vi "BMU诊断标定.vi"(5 "timeout":u32, 6 "Socket":dbl, 7 "通用配置?":bool, 8 "CAN端口":u16(ring), 9 "设备索引号":u16(ring), 10 "CAN卡类型":u32(ring)=21, 11 "从板号":u8=1) -> (3 "成功?":bool)   [LabVIEW 2013] (continued)
                                frame "电压起始值" {
                                n3880 = disable-structure shown="禁用" {
                                frame Disabled {
                                n3881 = local read "从板个数"() -> (w5557:dbl)
                                n3882 = Increment(x=w5557) -> (x+1=w5556:dbl)
                                n3883 = control-ref of="项目信息"() -> (w5563:refnum<vi>)
                                n3884 = for {
                                N: w5556 -> [_]
                                tunnel: [""] -> w5562 mode=indexing
                                }
                                n3885 = Multiply(x=u8 1, y=w5557) -> (x*y=w5559:dbl)
                                n3886 = Add(x=w5559, y=u8 21) -> (x+y=w5555:dbl)
                                n3887 = call "表格数据输入-8.6.vi"("行数"=w5555, "列数"=u32 1, "字符串数组"=w5562, "表格引用"=w5563) -> ()  [unwired: 8 in]
                                }
                                frame Enabled {
                                }
                                }
                                }
                                frame "温度个数" {
                                n3888 = local read "从板个数"() -> (w5567:dbl)
                                n3889 = Increment(x=w5567) -> (x+1=w5566:dbl)
                                n3890 = control-ref of="项目信息"() -> (w5573:refnum<vi>)
                                n3891 = for {
                                N: w5566 -> [_]
                                tunnel: [""] -> w5572 mode=indexing
                                }
                                n3892 = Multiply(x=u8 2, y=w5567) -> (x*y=w5569:dbl)
                                n3893 = Add(x=w5569, y=u8 22) -> (x+y=w5565:dbl)
                                n3894 = call "表格数据输入-8.6.vi"("行数"=w5565, "列数"=u32 1, "字符串数组"=w5572, "表格引用"=w5573) -> ()  [unwired: 8 in]
                                }
                                frame "温度起始值" {
                                n3895 = disable-structure shown="禁用" {
                                frame Disabled {
                                n3896 = local read "从板个数"() -> (w5577:dbl)
                                n3897 = Increment(x=w5577) -> (x+1=w5576:dbl)
                                n3898 = control-ref of="项目信息"() -> (w5583:refnum<vi>)
                                n3899 = for {
                                N: w5576 -> [_]
                                tunnel: [""] -> w5582 mode=indexing
                                }
                                n3900 = Multiply(x=u8 3, y=w5577) -> (x*y=w5579:dbl)
                                n3901 = Add(x=w5579, y=u8 23) -> (x+y=w5575:dbl)
                                n3902 = call "表格数据输入-8.6.vi"("行数"=w5575, "列数"=u32 1, "字符串数组"=w5582, "表格引用"=w5583) -> ()  [unwired: 8 in]
                                }
                                frame Enabled {
                                }
                                }
                                }
                                frame "保险位置" {
                                n3903 = local read "从板个数"() -> (w5587:dbl)
                                n3904 = control-ref of="项目信息"() -> (w5593:refnum<vi>)
                                n3905 = for {
                                N: 10 -> [_]
                                tunnel: [""] -> w5592 mode=indexing
                                }
                                n3906 = Multiply(x=u8 4, y=w5587) -> (x*y=w5589:dbl)
                                n3907 = Add(x=w5589, y=u8 24) -> (x+y=w5586:dbl)
                                n3908 = call "表格数据输入-8.6.vi"("行数"=w5586, "列数"=u32 1, "字符串数组"=w5592, "表格引用"=w5593) -> ()  [unwired: 8 in]
                                }
                                frame "电池额定实际容量" {
                                w5595 = 0.0 ("值")
                                n3909 = control-ref of="电池实际容量(A)"() -> (w5596:refnum<vi>)
                                n3910 = control-ref of="电池额定容量(A)"() -> (w5597:refnum<vi>)
                                n3911 = property class="DigNum (严格)"(reference=w5596, "Value"=w5595) -> ()  [unwired: 1 in, 2 out]
                                n3912 = property class="DigNum (严格)"(reference=w5597, "Value"=w5595) -> ()  [unwired: 1 in, 2 out]
                                }
                                frame "SOC" {
                                n3913 = control-ref of="SOC(%)"() -> (w5598:refnum<vi>)
                                n3914 = property class="DigNum (严格)"(reference=w5598, "Value"=0.0 ("值")) -> ()  [unwired: 1 in, 2 out]
                                }
                                frame "配置文件版本" {
                                n3915 = control-ref of="配置文件版本"() -> (w5600:refnum<vi>)
                                n3916 = property class="Str"(reference=w5600, "Value"="" ("值")) -> ()  [unwired: 1 in, 2 out]
                                }
                                frame "参数修改记录" {
                                n3917 = control-ref of="使用者"() -> (w5603:refnum<vi>)
                                n3918 = control-ref of="系统时钟"() -> (w5604:refnum<vi>)
                                n3919 = property class="DigNum (严格)"(reference=w5603, "Value"=0.0 ("值")) -> ()  [unwired: 1 in, 2 out]
                                n3920 = property class="Str"(reference=w5604, "Value"="" ("值")) -> ()  [unwired: 1 in, 2 out]
                                }
                                frame "校正时钟" {
                                n3921 = control-ref of="系统时钟"() -> (w5606:refnum<vi>)
                                n3922 = property class="Str"(reference=w5606, "Value"="" ("值")) -> ()  [unwired: 1 in, 2 out]
                                }
                                frame "车牌号" {
                                n3923 = control-ref of="车架(牌)号"() -> (w5608:refnum<vi>)
                                n3924 = property class="Str"(reference=w5608, "Value"="" ("值")) -> ()  [unwired: 1 in, 2 out]
                                }
                                frame "SOH" {
                                n3925 = control-ref of="SOH(%)"() -> (w5611:refnum<vi>)
                                n3926 = property class="DigNum (严格)"(reference=w5611, "Value"=0.0 ("值")) -> ()  [unwired: 1 in, 2 out]
                                }
                                frame "一级故障阀值" {
                                n3927 = local write "一级故障"(T10 {"总电压过高"=0.0, "整组电压不均衡"=0.0, "SOC过高"=0.0, "单体电压过高"=0.0, "总电压过低"=0.0, "温度过高"=0.0, "温度过低"=0.0, "单组电压不均衡"=0.0, "整组温度不均衡"=0.0, "单组温度不均衡"=0.0, "单体电压过低"=0.0, "充电电流过高"=0.0, "放电电流过高"=0.0, "SOC过低"=0.0, "内阻过大"=0.0, "极柱温度过高"=0.0, "SOH过低"=0.0} ("一级故障")) -> ()
                                }
                                frame "二级故障阀值" {
                                n3928 = local write "一级故障 2"(T10 {"总电压过高"=0.0, "整组电压不均衡"=0.0, "SOC过高"=0.0, "单体电压过高"=0.0, "总电压过低"=0.0, "温度过高"=0.0, "温度过低"=0.0, "单组电压不均衡"=0.0, "整组温度不均衡"=0.0, "单组温度不均衡"=0.0, "单体电压过低"=0.0, "充电电流过高"=0.0, "放电电流过高"=0.0, "SOC过低"=0.0, "内阻过大"=0.0, "极柱温度过高"=0.0, "SOH过低"=0.0} ("一级故障")) -> ()
                                }
                                frame "三级故障阀值" {
                                n3929 = local write "一级故障 3"(T10 {"总电压过高"=0.0, "整组电压不均衡"=0.0, "SOC过高"=0.0, "单体电压过高"=0.0, "总电压过低"=0.0, "温度过高"=0.0, "温度过低"=0.0, "单组电压不均衡"=0.0, "整组温度不均衡"=0.0, "单组温度不均衡"=0.0, "单体电压过低"=0.0, "充电电流过高"=0.0, "放电电流过高"=0.0, "SOC过低"=0.0, "内阻过大"=0.0, "极柱温度过高"=0.0, "SOH过低"=0.0} ("一级故障")) -> ()
                                }
                                frame "加热控制参数" {
                                n3930 = local write "加热控制参数"(T11 {"风机开启温度"=0.0, "风机关闭温度"=0.0, "加热开启温度"=0.0, "加热关闭温度"=0.0, "风机开启温差"=0.0, "风机关闭温差"=0.0, "加热关闭温差"=0.0} ("加热控制参数")) -> ()
                                }
                                frame "充电控制参数" {
                                n3931 = local write "一级故障 5"(T12 {"最大允许单体电压"=0.0, "最大允许总电压"=0.0, "最小允许单体电压"=0.0, "最大允许充电电流"=0.0, "最小允许充电电流"=0.0, "最大允许充电温度"=0.0, "最小允许充电温度"=0.0, "电流步长"=0.0} ("一级故障 5")) -> ()
                                }
                                frame "电池信息1" {
                                w5617 = ""
                                w5618 = 0.0 ("电池串联")
                                n3932 = local read "电池信息"() -> (w5620:T13)
                                n3933 = Bundle By Name(cluster=w5620, "电池串联"=w5618, "电池并联"=w5618, "电池包额定容量"=w5618, "电池包额定能量(kWh)"=w5618, "电池包额定总电压"=w5618, "实际容量"=w5618, "电池厂家"=w5617, "电池类型"=w5617, "电池生产日期"=w5617) -> (w5619:T13)
                                n3934 = local write "电池信息"(w5619) -> ()
                                }
                                frame "电池包组号" {
                                n3935 = local read "电池信息"() -> (w5623:T13)
                                n3936 = Bundle By Name(cluster=w5623, "电池包组号"="") -> (w5622:T13)
                                n3937 = local write "电池信息"(w5622) -> ()
                                }
                                frame "充放电安时" {
                                w5624 = 0.0 ("累计充电总安时")
                                n3938 = local read "电池信息"() -> (w5626:T13)
                                n3939 = Bundle By Name(cluster=w5626, "累计充电总安时"=w5624, "累计放电总安时"=w5624) -> (w5625:T13)
                                n3940 = local write "电池信息"(w5625) -> ()
                                }
                                frame "电池充放电次数" {
                                w5627 = 0.0 ("累计充电总安时")
                                n3941 = local read "电池信息"() -> (w5629:T13)
                                n3942 = Bundle By Name(cluster=w5629, "电池充满次数"=w5627, "电池放空次数"=w5627, "电池充电次数"=w5627) -> (w5628:T13)
                                n3943 = local write "电池信息"(w5628) -> ()
                                }
                                }
                              }
                              frame "从板" {
                                n3944 = case shown="\"温度起始值\"" w5630 {
                                frame "假", Default {
                                }
                                frame "电压起始值" {
                                n3945 = for {
                                N: 1 -> [_]
                                tunnel: [""] -> w5635 mode=indexing
                                }
                                n3946 = control-ref of="项目信息 2"() -> (w5631:refnum<vi>)
                                n3947 = call "表格数据输入-8.6.vi"("行数"=u32 0, "列数"=u32 1, "字符串数组"=w5635, "表格引用"=w5631) -> ()  [unwired: 8 in]
                                }
                                frame "通道电压个数" {
                                n3948 = for {
                                N: 5 -> [_]
                                tunnel: [""] -> w5641 mode=indexing
                                }
                                n3949 = control-ref of="项目信息 2"() -> (w5637:refnum<vi>)
                                n3950 = call "表格数据输入-8.6.vi"("行数"=u32 22, "列数"=u32 1, "字符串数组"=w5641, "表格引用"=w5637) -> ()  [unwired: 8 in]
                                }
                                frame "保险位置" {
                                n3951 = for {
                                N: 10 -> [_]
                                tunnel: [""] -> w5647 mode=indexing
                                }
                                n3952 = control-ref of="项目信息 2"() -> (w5643:refnum<vi>)
                                n3953 = call "表格数据输入-8.6.vi"("行数"=u32 2, "列数"=u32 1, "字符串数组"=w5647, "表格引用"=w5643) -> ()  [unwired: 8 in]
                                }
                                frame "温度起始值" {
                                n3954 = for {
                                N: 1 -> [_]
                                tunnel: [""] -> w5653 mode=indexing
                                }
                                n3955 = control-ref of="项目信息 2"() -> (w5649:refnum<vi>)
                                n3956 = call "表格数据输入-8.6.vi"("行数"=u32 1, "列数"=u32 1, "字符串数组"=w5653, "表格引用"=w5649) -> ()  [unwired: 8 in]
                                }
                                frame "加热控制参数" {
                                n3957 = local write "加热控制参数"(T11 {"风机开启温度"=0.0, "风机关闭温度"=0.0, "加热开启温度"=0.0, "加热关闭温度"=0.0, "风机开启温差"=0.0, "风机关闭温差"=0.0, "加热关闭温差"=0.0} ("加热控制参数")) -> ()
                                }
                                frame "一级故障阀值" {
                                n3958 = local write "一级故障 6"(T15 {"电压过高"=0.0, "电压过低"=0.0, "温度过高"=0.0, "温度过低"=0.0, "电压不均衡(V)"=0.0, "温度不均衡"=0.0, "SOC过低"=0.0} ("一级故障 6")) -> ()
                                }
                                frame "二级故障阀值" {
                                n3959 = local write "一级故障 7"(T15 {"电压过高"=0.0, "电压过低"=0.0, "温度过高"=0.0, "温度过低"=0.0, "电压不均衡(V)"=0.0, "温度不均衡"=0.0, "SOC过低"=0.0} ("一级故障 7")) -> ()
                                }
                                frame "三级故障阀值" {
                                n3960 = local write "一级故障 8"(T15 {"电压过高"=0.0, "电压过低"=0.0, "温度过高"=0.0, "温度过低"=0.0, "电压不均衡(V)"=0.0, "温度不均衡"=0.0, "SOC过低"=0.0} ("一级故障 7")) -> ()
                                }
                                frame "均衡参数" {
                                n3961 = local write "均衡参数"(T17 {"充电结束电压(90%)"=0.0, "充电结束电压(91%)"=0.0, "充电结束电压(92%)"=0.0, "充电结束电压(93%)"=0.0, "充电结束电压(94%)"=0.0, "均衡计算-电压高阀值1级"=0.0, "均衡计算-电压高阀值2级"=0.0, "均衡计算-电压低阀值1级"=0.0, "均衡计算-电压低阀值2级"=0.0, "均衡计算-最低电压阀值"=0.0, "均衡停止-最低电压阀值"=0.0, "均衡计算-电压极差阀值"=0.0, "充电结束电压(95%)"=0.0, "充电结束电压(96%)"=0.0, "充电结束电压(97%)"=0.0, "充电结束电压(98%)"=0.0, "充电结束电压(99%)"=0.0, "充电结束电压(100%)"=0.0} ("均衡参数")) -> ()
                                }
                                frame "均衡阀值" {
                                w5660 = sgl 0.0 ("均衡计算-电压高阀值1级")
                                n3962 = local read "均衡参数"() -> (w5661:T17)
                                n3963 = Bundle By Name(cluster=w5661, "均衡计算-电压高阀值1级"=w5660, "均衡计算-电压高阀值2级"=w5660, "均衡计算-电压低阀值1级"=w5660, "均衡计算-电压低阀值2级"=w5660, "均衡计算-最低电压阀值"=w5660, "均衡停止-最低电压阀值"=w5660, "均衡计算-电压极差阀值"=w5660) -> (w5662:T17)
                                n3964 = local write "均衡参数"(w5662) -> ()
                                }
                                frame "充电结束电压" {
                                w5663 = sgl 0.0 ("均衡计算-电压高阀值1级")
                                n3965 = local read "均衡参数"() -> (w5664:T17)
                                n3966 = Bundle By Name(cluster=w5664, "充电结束电压(90%)"=w5663, "充电结束电压(91%)"=w5663, "充电结束电压(92%)"=w5663, "充电结束电压(93%)"=w5663, "充电结束电压(94%)"=w5663, "充电结束电压(95%)"=w5663, "充电结束电压(96%)"=w5663, "充电结束电压(97%)"=w5663, "充电结束电压(98%)"=w5663, "充电结束电压(99%)"=w5663, "充电结束电压(100%)"=w5663) -> (w5665:T17)
                                n3967 = local write "均衡参数"(w5665) -> ()
                                }
                                }
                              }
                            }
                          }
                          frame #1 {
                            w5666 = FALSE ("流控帧")
                            w5667 = TRUE ("流控帧 2")
                            n3968 = global write "EV05全局变量1.vi" "写入超时"(w5666) -> ()
                            n3969 = global write "EV05全局变量1.vi" "流控帧"(w5666) -> ()
                            n3970 = local write "写?"(w5666) -> ()
                            n3971 = local write "消除"(w5667) -> ()
                            n3972 = local write "控制1"(w5667) -> ()
                            n3973 = global write "EV05全局变量1.vi" "流控帧 2"(w5667) -> ()
                          }
                          frame #2 {
                            n3974 = Wait Until Next ms Multiple(millisecond multiple=u32 300 ("毫秒倍数")) -> ()  [unwired: 1 out]
                          }
                          frame #3 {
                            n3975 = local read "设备索引号"() -> (w5670:u16)
                            n3976 = local read "CAN卡类型"() -> (w5671:u32)
                            n3977 = local read "CAN端口"() -> (w5669:u16)
                            n3978 = local write "命令序号"(w5674) -> ()
                            n3979 = stacked-sequence {
                              tunnel: w5675 -> [_ w5682]
                              tunnel: w5674 -> [_ w5681]
                              tunnel: w5673 -> [_ w5680]
                              tunnel: w5672 -> [_ w5679]
                              tunnel: w5671 -> [_ w5678]
                              tunnel: w5670 -> [_ w5677]
                              tunnel: w5669 -> [_ w5676]
                              frame #0 {
                              }
                              frame #1 {
                                n3980 = call "多帧发送机制(EV05).vi"("can卡类型"=w5678, "设备索引号"=w5677, "CAN端口"=w5676, "命令"=w5682, "板号"=w5680, "命令序号"=w5681, "输入数据"=w5679) -> ()  [unwired: 2 in, 11 out]
                              }
                            }
                          }
                          frame #4 {
                            n3981 = while {
                              tunnel: [w5687] -> w5684
                              tunnel: [w5686] -> w5683
                              i -> [w5690]
                              stop <- w5687 stop-if-true
                              n3982 = local read "强制终止读写标记"() -> (w5685:bool)
                              n3983 = global read "EV05全局变量1.vi" "写入超时"() -> (w5686:bool)
                              n3984 = Greater Or Equal?(x=w5690, y=20) -> (x >= y?=w5688:bool)
                              n3985 = Compound Arithmetic op=OR(w5685, w5686, w5688) -> (w5687:bool)
                              n3986 = Wait Until Next ms Multiple(millisecond multiple=u32 100 ("毫秒倍数")) -> ()  [unwired: 1 out]
                            }
                          }
                          frame #5 {
                            n3987 = case shown="假" w5699 {
                              tunnel: w5698 -> [w5710 _]
                              tunnel: [w5705 w5722] -> w5697
                              tunnel: w5696 -> [w5704 _]
                              tunnel: w5695 -> [w5703 w5722]
                              tunnel: [w5702 w5721] -> w5692
                              tunnel: w5694 -> [w5701 _]
                              tunnel: w5693 -> [w5700 w5721]
                              frame False {
                                n3988 = local read "重试次数"() -> (w5709:u8)
                                n3989 = Increment(x=w5709) -> (x+1=w5708:u8)
                                n3990 = Greater Or Equal?(x=w5708, y=u8 4) -> (x >= y?=w5707:bool)
                                n3991 = local write "重试次数"(w5708) -> ()
                                n3992 = case shown="真" w5707 {
                                tunnel: w5710 -> [_ w5715]
                                tunnel: [w5712 w5714] -> w5705
                                tunnel: w5704 -> [w5712 _]
                                tunnel: w5703 -> [_ w5714]
                                tunnel: [w5711 w5713] -> w5702
                                tunnel: w5701 -> [w5711 _]
                                tunnel: w5700 -> [_ w5713]
                                frame False {
                                }
                                frame True {
                                n3993 = control-ref of="结果"() -> (w5717:refnum<vi>)
                                n3994 = Concatenate Strings(w5715, "     读取失败" ("字符串")) -> (w5719:string)
                                n3995 = Build Array(w5719) -> (w5716:string[])
                                n3996 = call "表格编辑.vi"("新元素/子数组"=w5716, "活动单元格:单元格背景色"=u32 16740749, "MCListbox引用句柄"=w5717) -> ()  [unwired: 9 out]
                                }
                                }
                              }
                              frame True {
                              }
                            }
                          }
                          frame #6 {
                            n3997 = And(x=w5724, y=w5726) -> (x .and. y?=w5725:bool)
                            n3998 = case shown="真" w5725 {
                              frame False {
                              }
                              frame True {
                                n3999 = local write "强制终止读写标记"(FALSE ("强制停止")) -> ()
                                n4000 = control-ref of="结果"() -> (w5729:refnum<vi>)
                                n4001 = Concatenate Strings("读取完成" ("字符串")) -> (w5731:string)
                                n4002 = Build Array(w5731) -> (w5728:string[])
                                n4003 = call "表格编辑.vi"("新元素/子数组"=w5728, "活动单元格:单元格背景色"=u32 21937, "MCListbox引用句柄"=w5729) -> ()  [unwired: 9 out]
                              }
                            }
                            n4004 = Wait (ms)(milliseconds to wait=u32 50 ("等待时间（毫秒）")) -> ()  [unwired: 1 out]
                          }
                        }
                      }
                    }
                  }
                  n4005 = local read "强制终止读写标记"() -> (w5497:bool)
                  n4006 = Or(x=w5497, y=w5496) -> (x .or. y?=w5494:bool)
                }
              }
            }
            frame #2 {
              n4007 = case shown="假" w5816 {
                tunnel: w5817 -> [w5818 _]
                frame False {
                  n4008 = case shown="\"主板\", 默认" w5818 {
                    frame "主板", Default {
                      n4009 = global read "读配置文件全局.vi" "电池额定实际容量判定"() -> (w5832:bool)
                      n4010 = global read "读配置文件全局.vi" "电池充放电次数判定"() -> (w5821:bool)
                      n4011 = global read "读配置文件全局.vi" "加热控制参数判定"() -> (w5819:bool)
                      n4012 = global read "读配置文件全局.vi" "配置文件版本判定"() -> (w5831:bool)
                      n4013 = global read "读配置文件全局.vi" "充电控制参数判定"() -> (w5825:bool)
                      n4014 = global read "读配置文件全局.vi" "通道电压数判定"() -> (w5837:bool)
                      n4015 = global read "读配置文件全局.vi" "电压起始值判定"() -> (w5836:bool)
                      n4016 = global read "读配置文件全局.vi" "温度起始值判定"() -> (w5834:bool)
                      n4017 = global read "读配置文件全局.vi" "充放电安时判定"() -> (w5823:bool)
                      n4018 = global read "读配置文件全局.vi" "电池包组号判定"() -> (w5822:bool)
                      n4019 = global read "读配置文件全局.vi" "电池信息1判定"() -> (w5824:bool)
                      n4020 = global read "读配置文件全局.vi" "从板个数判定"() -> (w5840:bool)
                      n4021 = global read "读配置文件全局.vi" "产品编号判定"() -> (w5839:bool)
                      n4022 = global read "读配置文件全局.vi" "电压个数判定"() -> (w5838:bool)
                      n4023 = global read "读配置文件全局.vi" "温度个数判定"() -> (w5835:bool)
                      n4024 = global read "读配置文件全局.vi" "保险位置判定"() -> (w5833:bool)
                      n4025 = global read "读配置文件全局.vi" "一级故障判定"() -> (w5828:bool)
                      n4026 = global read "读配置文件全局.vi" "二级故障判定"() -> (w5827:bool)
                      n4027 = global read "读配置文件全局.vi" "三级故障判定"() -> (w5826:bool)
                      n4028 = global read "读配置文件全局.vi" "车牌号判定"() -> (w5830:bool)
                      n4029 = global read "读配置文件全局.vi" "SOH判定"() -> (w5829:bool)
                      n4030 = Build Array(w5840, w5839, w5838, w5837, w5836, w5835, w5834, w5833, w5832, w5831, w5830, w5829, w5828, w5827, w5826, w5825, w5824, w5823, w5822, w5821, w5819) -> (w5820:bool[])
                      n4031 = And Array Elements(Boolean array=w5820) -> (logical AND=w5841:bool)
                      n4032 = disable-structure shown="禁用" {
                        frame Disabled {
                          n4033 = global read "读配置文件全局.vi" "SOC判定"() -> ()  [unwired: 1 out]
                        }
                        frame Enabled {
                        }
                      }
                      n4034 = case shown="假" w5841 {
                        tunnel: w5820 -> [_ w5846]
                        frame True {
                          n4035 = control-ref of="结果"() -> (w5844:refnum<vi>)
                          n4036 = Build Array("全部判定成功!!!!!!!!") -> (w5845:string[])
                          n4037 = call "表格编辑.vi"("新元素/子数组"=w5845, "活动单元格:单元格背景色"=u32 6618880, "MCListbox引用句柄"=w5844) -> ()  [unwired: 9 out]
                        }
                        frame False {
                          n4038 = stacked-sequence {
                            tunnel: w5846 -> [_ w5851]
                            frame #0 {
                              n4039 = control-ref of="结果"() -> (w5849:refnum<vi>)
                              n4040 = Build Array("全部判定失败!!!!!") -> (w5850:string[])
                              n4041 = call "表格编辑.vi"("新元素/子数组"=w5850, "活动单元格:单元格背景色"=u32 16711680, "MCListbox引用句柄"=w5849) -> ()  [unwired: 9 out]
                            }
                            frame #1 {
                              n4042 = for {
                                tunnel: w5851 -> [w5853] mode=indexing
                                i -> [w5852]
                                n4043 = case shown="20" w5852 {
                                tunnel: w5853 -> [w5854 w5859 w5864 w5869 w5874 w5879 w5884 w5889 w5894 w5899 w5904 w5909 w5914 w5919 w5924 w5929 w5934 w5939 w5944 w5949 w5954 _]
                                frame 0 {
                                n4044 = case shown="假" w5854 {
                                frame False {
                                n4045 = control-ref of="结果"() -> (w5857:refnum<vi>)
                                n4046 = Build Array("从板个数判定失败!") -> (w5858:string[])
                                n4047 = call "表格编辑.vi"("新元素/子数组"=w5858, "活动单元格:单元格背景色"=u32 16711680, "MCListbox引用句柄"=w5857) -> ()  [unwired: 9 out]
                                }
                                frame True {
                                }
                                }
                                }
                                frame 1 {
                                n4048 = case shown="假" w5859 {
                                frame False {
                                n4049 = control-ref of="结果"() -> (w5862:refnum<vi>)
                                n4050 = Build Array("产品编号判定失败!") -> (w5863:string[])
                                n4051 = call "表格编辑.vi"("新元素/子数组"=w5863, "活动单元格:单元格背景色"=u32 16711680, "MCListbox引用句柄"=w5862) -> ()  [unwired: 9 out]
                                }
                                frame True {
                                }
                                }
                                }
                                frame 2 {
                                n4052 = case shown="假" w5864 {
                                frame False {
                                n4053 = control-ref of="结果"() -> (w5867:refnum<vi>)
                                n4054 = Build Array("电压个数判定失败!") -> (w5868:string[])
                                n4055 = call "表格编辑.vi"("新元素/子数组"=w5868, "活动单元格:单元格背景色"=u32 16711680, "MCListbox引用句柄"=w5867) -> ()  [unwired: 9 out]
                                }
                                frame True {
                                }
                                }
                                }
                                frame 3 {
                                n4056 = case shown="假" w5869 {
                                frame False {
                                n4057 = control-ref of="结果"() -> (w5872:refnum<vi>)
                                n4058 = Build Array("通道电压数判定失败!") -> (w5873:string[])
                                n4059 = call "表格编辑.vi"("新元素/子数组"=w5873, "活动单元格:单元格背景色"=u32 16711680, "MCListbox引用句柄"=w5872) -> ()  [unwired: 9 out]
                                }
                                frame True {
                                }
                                }
                                }
                                frame 4 {
                                n4060 = case shown="假" w5874 {
                                frame False {
                                n4061 = control-ref of="结果"() -> (w5877:refnum<vi>)
                                n4062 = Build Array("电压起始值判定失败!") -> (w5878:string[])
                                n4063 = call "表格编辑.vi"("新元素/子数组"=w5878, "活动单元格:单元格背景色"=u32 16711680, "MCListbox引用句柄"=w5877) -> ()  [unwired: 9 out]
                                }
                                frame True {
                                }
                                }
                                }
                                frame 5 {
                                n4064 = case shown="假" w5879 {
                                frame False {
                                n4065 = control-ref of="结果"() -> (w5882:refnum<vi>)
                                n4066 = Build Array("温度个数判定失败!") -> (w5883:string[])
                                n4067 = call "表格编辑.vi"("新元素/子数组"=w5883, "活动单元格:单元格背景色"=u32 16711680, "MCListbox引用句柄"=w5882) -> ()  [unwired: 9 out]
                                }
                                frame True {
                                }
                                }
                                }
                                frame 6 {
                                n4068 = case shown="假" w5884 {
                                frame False {
                                n4069 = control-ref of="结果"() -> (w5887:refnum<vi>)
                                n4070 = Build Array("温度起始值判定失败!") -> (w5888:string[])
                                n4071 = call "表格编辑.vi"("新元素/子数组"=w5888, "活动单元格:单元格背景色"=u32 16711680, "MCListbox引用句柄"=w5887) -> ()  [unwired: 9 out]
                                }
                                frame True {
                                }
                                }
                                }
                                frame 7 {
                                n4072 = case shown="假" w5889 {
                                frame False {
                                n4073 = control-ref of="结果"() -> (w5892:refnum<vi>)
                                n4074 = Build Array("保险位置判定失败!") -> (w5893:string[])
                                n4075 = call "表格编辑.vi"("新元素/子数组"=w5893, "活动单元格:单元格背景色"=u32 16711680, "MCListbox引用句柄"=w5892) -> ()  [unwired: 9 out]
                                }
                                frame True {
                                }
                                }
                                }
                                frame 8 {
                                n4076 = case shown="假" w5894 {
                                frame False {
                                n4077 = control-ref of="结果"() -> (w5897:refnum<vi>)
                                n4078 = Build Array("电池额定实际容量判定失败!") -> (w5898:string[])
                                n4079 = call "表格编辑.vi"("新元素/子数组"=w5898, "活动单元格:单元格背景色"=u32 16711680, "MCListbox引用句柄"=w5897) -> ()  [unwired: 9 out]
                                }
                                frame True {
                                }
                                }
                                }
                                frame 9 {
                                n4080 = case shown="假" w5899 {
                                frame False {
                                n4081 = control-ref of="结果"() -> (w5902:refnum<vi>)
                                n4082 = Build Array("配置文件版本判定失败!") -> (w5903:string[])
                                n4083 = call "表格编辑.vi"("新元素/子数组"=w5903, "活动单元格:单元格背景色"=u32 16711680, "MCListbox引用句柄"=w5902) -> ()  [unwired: 9 out]
                                }
                                frame True {
                                }
                                }
                                }
                                frame 10 {
                                n4084 = case shown="假" w5904 {
                                frame False {
                                n4085 = control-ref of="结果"() -> (w5907:refnum<vi>)
                                n4086 = Build Array("车牌号判定失败!") -> (w5908:string[])
                                n4087 = call "表格编辑.vi"("新元素/子数组"=w5908, "活动单元格:单元格背景色"=u32 16711680, "MCListbox引用句柄"=w5907) -> ()  [unwired: 9 out]
                                }
                                frame True {
                                }
                                }
                                }
                                frame 11 {
                                n4088 = case shown="假" w5909 {
                                frame False {
                                n4089 = control-ref of="结果"() -> (w5912:refnum<vi>)
                                n4090 = Build Array("SOH判定失败!") -> (w5913:string[])
                                n4091 = call "表格编辑.vi"("新元素/子数组"=w5913, "活动单元格:单元格背景色"=u32 16711680, "MCListbox引用句柄"=w5912) -> ()  [unwired: 9 out]
                                }
                                frame True {
                                }
                                }
                                }
                                frame 12 {
                                n4092 = case shown="假" w5914 {
                                frame False {
                                n4093 = control-ref of="结果"() -> (w5917:refnum<vi>)
                                n4094 = Build Array("一级故障阀值判定失败!") -> (w5918:string[])
                                n4095 = call "表格编辑.vi"("新元素/子数组"=w5918, "活动单元格:单元格背景色"=u32 16711680, "MCListbox引用句柄"=w5917) -> ()  [unwired: 9 out]
                                }
                                frame True {
                                }
                                }
                                }
                                frame 13 {
                                n4096 = case shown="假" w5919 {
                                frame False {
                                n4097 = control-ref of="结果"() -> (w5922:refnum<vi>)
                                n4098 = Build Array("二级故障阀值判定失败!") -> (w5923:string[])
                                n4099 = call "表格编辑.vi"("新元素/子数组"=w5923, "活动单元格:单元格背景色"=u32 16711680, "MCListbox引用句柄"=w5922) -> ()  [unwired: 9 out]
                                }
                                frame True {
                                }
                                }
                                }
                                frame 14 {
                                n4100 = case shown="假" w5924 {
                                frame False {
                                n4101 = control-ref of="结果"() -> (w5927:refnum<vi>)
                                n4102 = Build Array("三级故障阀值判定失败!") -> (w5928:string[])
                                n4103 = call "表格编辑.vi"("新元素/子数组"=w5928, "活动单元格:单元格背景色"=u32 16711680, "MCListbox引用句柄"=w5927) -> ()  [unwired: 9 out]
                                }
                                frame True {
                                }
                                }
                                }
                                frame 15 {
                                n4104 = case shown="假" w5929 {
                                frame False {
                                n4105 = control-ref of="结果"() -> (w5932:refnum<vi>)
                                n4106 = Build Array("充电控制参数判定失败!") -> (w5933:string[])
                                n4107 = call "表格编辑.vi"("新元素/子数组"=w5933, "活动单元格:单元格背景色"=u32 16711680, "MCListbox引用句柄"=w5932) -> ()  [unwired: 9 out]
                                }
                                frame True {
                                }
                                }
                                }
                                frame 16 {
                                n4108 = case shown="假" w5934 {
                                frame False {
                                n4109 = control-ref of="结果"() -> (w5937:refnum<vi>)
                                n4110 = Build Array("电池信息1判定失败!") -> (w5938:string[])
                                n4111 = call "表格编辑.vi"("新元素/子数组"=w5938, "活动单元格:单元格背景色"=u32 16711680, "MCListbox引用句柄"=w5937) -> ()  [unwired: 9 out]
                                }
                                frame True {
                                }
                                }
                                }
                                frame 17 {
                                n4112 = case shown="假" w5939 {
                                frame False {
                                n4113 = control-ref of="结果"() -> (w5942:refnum<vi>)
                                n4114 = Build Array("充放电安时判定失败!") -> (w5943:string[])
                                n4115 = call "表格编辑.vi"("新元素/子数组"=w5943, "活动单元格:单元格背景色"=u32 16711680, "MCListbox引用句柄"=w5942) -> ()  [unwired: 9 out]
                                }
                                frame True {
                                }
                                }
                                }
                                frame 18 {
                                n4116 = case shown="假" w5944 {
                                frame False {
                                n4117 = control-ref of="结果"() -> (w5947:refnum<vi>)
                                n4118 = Build Array("电池包组号判定失败!") -> (w5948:string[])
                                n4119 = call "表格编辑.vi"("新元素/子数组"=w5948, "活动单元格:单元格背景色"=u32 16711680, "MCListbox引用句柄"=w5947) -> ()  [unwired: 9 out]
                                }
                                frame True {
                                }
                                }
                                }
                                frame 19 {
                                n4120 = case shown="假" w5949 {
                                frame False {
                                n4121 = control-ref of="结果"() -> (w5952:refnum<vi>)
                                n4122 = Build Array("电池充放电次数判定失败!") -> (w5953:string[])
                                n4123 = call "表格编辑.vi"("新元素/子数组"=w5953, "活动单元格:单元格背景色"=u32 16711680, "MCListbox引用句柄"=w5952) -> ()  [unwired: 9 out]
                                }
                                frame True {
                                }
                                }
                                }
                                frame 20 {
                                n4124 = case shown="假" w5954 {
                                frame False {
                                n4125 = control-ref of="结果"() -> (w5957:refnum<vi>)
                                n4126 = Build Array("加热控制参数判定失败!") -> (w5958:string[])
                                n4127 = call "表格编辑.vi"("新元素/子数组"=w5958, "活动单元格:单元格背景色"=u32 16711680, "MCListbox引用句柄"=w5957) -> ()  [unwired: 9 out]
                                }
                                frame True {
                                }
                                }
                                }
                                frame 99, Default {
                                }
                                }
                              }
                            }
                          }
                        }
                      }
                    }
                    frame "从板" {
                      n4128 = global read "读配置文件全局2.vi" "电压起始值判定"() -> (w5967:bool)
                      n4129 = global read "读配置文件全局2.vi" "温度起始值判定"() -> (w5964:bool)
                      n4130 = global read "读配置文件全局2.vi" "加热控制参数判定"() -> (w5959:bool)
                      n4131 = global read "读配置文件全局2.vi" "通道电压判定"() -> (w5966:bool)
                      n4132 = global read "读配置文件全局2.vi" "保险位置判定"() -> (w5965:bool)
                      n4133 = global read "读配置文件全局2.vi" "一级故障判定"() -> (w5962:bool)
                      n4134 = global read "读配置文件全局2.vi" "二级故障判定"() -> (w5961:bool)
                      n4135 = global read "读配置文件全局2.vi" "三级故障判定"() -> (w5960:bool)
                      n4136 = global read "读配置文件全局2.vi" "从板号判定"() -> (w5968:bool)
                      n4137 = Build Array(w5968, w5967, w5966, w5965, w5964, w5962, w5961, w5960, w5959) -> (w5963:bool[])
                      n4138 = And Array Elements(Boolean array=w5963) -> (logical AND=w5969:bool)
                      n4139 = case shown="假" w5969 {
                        tunnel: w5963 -> [_ w5974]
                        frame True {
                          n4140 = control-ref of="结果"() -> (w5972:refnum<vi>)
                          n4141 = Build Array("读取判定成功!!!!!!!!") -> (w5973:string[])
                          n4142 = call "表格编辑.vi"("新元素/子数组"=w5973, "活动单元格:单元格背景色"=u32 6618880, "MCListbox引用句柄"=w5972) -> ()  [unwired: 9 out]
                        }
                        frame False {
                          n4143 = stacked-sequence {
                            tunnel: w5974 -> [_ w5979]
                            frame #0 {
                              n4144 = control-ref of="结果"() -> (w5977:refnum<vi>)
                              n4145 = Build Array("读取判定失败!!!!!") -> (w5978:string[])
                              n4146 = call "表格编辑.vi"("新元素/子数组"=w5978, "活动单元格:单元格背景色"=u32 16711680, "MCListbox引用句柄"=w5977) -> ()  [unwired: 9 out]
                            }
                            frame #1 {
                              n4147 = for {
                                tunnel: w5979 -> [w5980] mode=indexing
                                i -> [w5981]
                                n4148 = case shown="0" w5981 {
                                tunnel: w5980 -> [w5982 w5987 w5992 w5997 w6002 w6007 w6012 w6017 w6022 _]
                                frame 0 {
                                n4149 = case shown="假" w5982 {
                                frame False {
                                n4150 = control-ref of="结果"() -> (w5985:refnum<vi>)
                                n4151 = Build Array("从板号判定失败!") -> (w5986:string[])
                                n4152 = call "表格编辑.vi"("新元素/子数组"=w5986, "活动单元格:单元格背景色"=u32 16711680, "MCListbox引用句柄"=w5985) -> ()  [unwired: 9 out]
                                }
                                frame True {
                                }
                                }
                                }
                                frame 1 {
                                n4153 = case shown="假" w5987 {
                                frame False {
                                n4154 = control-ref of="结果"() -> (w5990:refnum<vi>)
                                n4155 = Build Array("电压起始值判定失败!") -> (w5991:string[])
                                n4156 = call "表格编辑.vi"("新元素/子数组"=w5991, "活动单元格:单元格背景色"=u32 16711680, "MCListbox引用句柄"=w5990) -> ()  [unwired: 9 out]
                                }
                                frame True {
                                }
                                }
                                }
                                frame 2 {
                                n4157 = case shown="假" w5992 {
                                frame False {
                                n4158 = control-ref of="结果"() -> (w5995:refnum<vi>)
                                n4159 = Build Array("通道电压节数判定失败!") -> (w5996:string[])
                                n4160 = call "表格编辑.vi"("新元素/子数组"=w5996, "活动单元格:单元格背景色"=u32 16711680, "MCListbox引用句柄"=w5995) -> ()  [unwired: 9 out]
                                }
                                frame True {
                                }
                                }
                                }
                                frame 3 {
                                n4161 = case shown="假" w5997 {
                                frame False {
                                n4162 = control-ref of="结果"() -> (w6000:refnum<vi>)
                                n4163 = Build Array("保险位置判定失败!") -> (w6001:string[])
                                n4164 = call "表格编辑.vi"("新元素/子数组"=w6001, "活动单元格:单元格背景色"=u32 16711680, "MCListbox引用句柄"=w6000) -> ()  [unwired: 9 out]
                                }
                                frame True {
                                }
                                }
                                }
                                frame 4 {
                                n4165 = case shown="假" w6002 {
                                frame False {
                                n4166 = control-ref of="结果"() -> (w6005:refnum<vi>)
                                n4167 = Build Array("温度起始值判定失败!") -> (w6006:string[])
                                n4168 = call "表格编辑.vi"("新元素/子数组"=w6006, "活动单元格:单元格背景色"=u32 16711680, "MCListbox引用句柄"=w6005) -> ()  [unwired: 9 out]
                                }
                                frame True {
                                }
                                }
                                }
                                frame 5 {
                                n4169 = case shown="假" w6007 {
                                frame False {
                                n4170 = control-ref of="结果"() -> (w6010:refnum<vi>)
                                n4171 = Build Array("一级故障判定失败!") -> (w6011:string[])
                                n4172 = call "表格编辑.vi"("新元素/子数组"=w6011, "活动单元格:单元格背景色"=u32 16711680, "MCListbox引用句柄"=w6010) -> ()  [unwired: 9 out]
                                }
                                frame True {
                                }
                                }
                                }
                                frame 6 {
                                n4173 = case shown="假" w6012 {
                                frame False {
                                n4174 = control-ref of="结果"() -> (w6015:refnum<vi>)
                                n4175 = Build Array("二级故障判定失败!") -> (w6016:string[])
                                n4176 = call "表格编辑.vi"("新元素/子数组"=w6016, "活动单元格:单元格背景色"=u32 16711680, "MCListbox引用句柄"=w6015) -> ()  [unwired: 9 out]
                                }
                                frame True {
                                }
                                }
                                }
                                frame 7 {
                                n4177 = case shown="假" w6017 {
                                frame False {
                                n4178 = control-ref of="结果"() -> (w6020:refnum<vi>)
                                n4179 = Build Array("三级故障判定失败!") -> (w6021:string[])
                                n4180 = call "表格编辑.vi"("新元素/子数组"=w6021, "活动单元格:单元格背景色"=u32 16711680, "MCListbox引用句柄"=w6020) -> ()  [unwired: 9 out]
                                }
                                frame True {
                                }
                                }
                                }
                                frame 8 {
                                n4181 = case shown="假" w6022 {
                                frame False {
                                n4182 = control-ref of="结果"() -> (w6025:refnum<vi>)
                                n4183 = Build Array("加热控制参数判定失败!") -> (w6026:string[])
                                n4184 = call "表格编辑.vi"("新元素/子数组"=w6026, "活动单元格:单元格背景色"=u32 16711680, "MCListbox引用句柄"=w6025) -> ()  [unwired: 9 out]
                                }
                                frame True {
                                }
                                }
                                }
                                frame 99, Default {
                                }
                                }
                              }
                            }
                          }
                        }
                      }
                      n4185 = disable-structure shown="禁用" {
                        frame Disabled {
                          n4186 = global read "读配置文件全局.vi" "SOC判定"() -> ()  [unwired: 1 out]
                        }
                        frame Enabled {
                        }
                      }
                    }
                  }
                }
                frame True {
                }
              }
            }
          }
          n4187 = stacked-sequence {
            tunnel: w5259 -> [_]
            frame #0 {
              n4188 = local write "强制终止读写标记"(FALSE ("强制停止")) -> ()
            }
          }
          "重试次数" <- u8 0 ("重试次数")
        }
        frame "开启均衡" {
          n4189 = local read "从板板号"() -> (w6027:u8)
          n4190 = stacked-sequence {
            tunnel: 133 -> [_ w6053 _ _]
            tunnel: w6027 -> [_ _ _ _]
            frame #0 {
              w6037 = u8 0 items=["Normal", "Listen Only"] ("工作方式")
              w6036 = u8 1 items=["Dual Filter", "Single Filter"] ("滤波方式")
              n4191 = global write "EV05全局变量1.vi" "读取超时"(FALSE ("读取超时")) -> ()
              n4192 = global write "EV05全局变量1.vi" "流控帧 2"(TRUE ("流控帧 2")) -> ()
              n4193 = local write "写?"(TRUE ("写?")) -> ()
              n4194 = local read "设备索引号"() -> (w6032:u16)
              n4195 = local read "CAN卡类型"() -> (w6031:u32)
              n4196 = local read "CAN端口"() -> (w6033:u16)
              n4197 = local write "控制1"(TRUE ("控制1")) -> ()
              n4198 = local write "消除"(TRUE ("消除")) -> ()
              n4199 = global write "EV05全局变量1.vi" "流控帧"(FALSE ("流控帧")) -> ()
              n4200 = call "CAN_Init-8.6.vi"("CAN卡类型"=w6031, "设备索引号"=w6032, "CAN端口"=w6033, "操作类型"=enum16{"初始化CAN", "关闭CAN"}."初始化CAN", "滤波方式"=w6036, "Accept Code"=u32 606601216, "簇"=T23 {"打开CAN"=FALSE, "初始化CAN"=TRUE, "开始CAN"=TRUE, "重启"=FALSE, "关闭CAN"=FALSE}, "Mask Code"=u32 524287 ("Accept Code"), "工作方式"=w6037, "是否滤波"=TRUE, "滤波选择"=T22 {"fiter_mode"=1, "fiter_endid"=75825152, "fiter_startid"=75890687}) -> ()  [unwired: 3 in, 6 out]
              n4201 = Wait Until Next ms Multiple(millisecond multiple=u32 20 ("毫秒倍数")) -> ()  [unwired: 1 out]
            }
            frame #1 {
              n4202 = local write "命令"(w6053) -> ()
              n4203 = call "ID组合.vi"("SA(4)"=0 ("PDU(1)"), "PS(3)"=63 ("PDU(1)"), "PF(2)"=w6053, "PDU(1)"=4) -> ("ID"=w6052:i32)  [unwired: 7 out]
              n4204 = local read "均衡类型选择"() -> (w6049:enum16{"放电均衡", "充电均衡", "充放电均衡"})
              n4205 = local read "设备索引号"() -> (w6058:u16)
              n4206 = local read "CAN卡类型"() -> (w6059:u32)
              n4207 = local read "CAN端口"() -> (w6057:u16)
              n4208 = local write "命令序号"(2) -> ()
              n4209 = Add(x=w6049, y=1) -> (x+y=w6047:i32)
              n4210 = Build Array(2, 2, w6047) -> (w6060:i32[])
              n4211 = call "transmit-8.6.vi"("can卡类型"=w6059, "设备索引号"=w6058, "CAN端口"=w6057, "ID"=w6052, "SendType"=u8 0, "Data"=w6060) -> ()  [unwired: 3 in, 11 out]
            }
            frame #2 {
              n4212 = Wait Until Next ms Multiple(millisecond multiple=u32 1000 ("毫秒倍数")) -> ()  [unwired: 1 out]
            }
            frame #3 {
              w6068 = u8 0 items=["Normal", "Listen Only"] ("工作方式")
              w6069 = u8 1 items=["Dual Filter", "Single Filter"] ("滤波方式")
              n4213 = global write "EV05全局变量1.vi" "流控帧 2"(FALSE ("流控帧 2")) -> ()
              n4214 = local read "CAN卡类型"() -> (w6074:u32)
              n4215 = local read "设备索引号"() -> (w6073:u16)
              n4216 = local read "CAN端口"() -> (w6072:u16)
              n4217 = local write "控制1"(FALSE ("控制1")) -> ()
              n4218 = local write "消除"(FALSE ("消除")) -> ()
              n4219 = call <vilib>:"Unset Busy.vi"() -> ()  [unwired: 2 in, 10 out]
              n4220 = call "CAN_Init-8.6.vi"("CAN卡类型"=w6074, "设备索引号"=w6073, "CAN端口"=w6072, "操作类型"=enum16{"初始化CAN", "关闭CAN"}."初始化CAN", "滤波方式"=w6069, "Accept Code"=u32 3221225472, "簇"=T23 {"打开CAN"=FALSE, "初始化CAN"=TRUE, "开始CAN"=TRUE, "重启"=FALSE, "关闭CAN"=FALSE}, "Mask Code"=u32 1073741823 ("Accept Code"), "工作方式"=w6068, "是否滤波"=TRUE, "滤波选择"=T22 {"fiter_mode"=1, "fiter_endid"=402653184, "fiter_startid"=419430399}) -> ()  [unwired: 3 in, 6 out]
            }
          }
        }
        frame "关闭均衡" {
          n4221 = local read "从板板号"() -> (w6078:u8)
          n4222 = stacked-sequence {
            tunnel: 133 -> [_ w6102 _ _]
            tunnel: w6078 -> [_ _ _ _]
            frame #0 {
              w6088 = u8 0 items=["Normal", "Listen Only"] ("工作方式")
              w6087 = u8 1 items=["Dual Filter", "Single Filter"] ("滤波方式")
              n4223 = global write "EV05全局变量1.vi" "读取超时"(FALSE ("读取超时")) -> ()
              n4224 = global write "EV05全局变量1.vi" "流控帧 2"(TRUE ("流控帧 2")) -> ()
              n4225 = local write "写?"(TRUE ("写?")) -> ()
              n4226 = local read "设备索引号"() -> (w6083:u16)
              n4227 = local read "CAN卡类型"() -> (w6082:u32)
              n4228 = local read "CAN端口"() -> (w6084:u16)
              n4229 = local write "控制1"(TRUE ("控制1")) -> ()
              n4230 = global write "EV05全局变量1.vi" "流控帧"(FALSE ("流控帧")) -> ()
              n4231 = local write "消除"(TRUE ("消除")) -> ()
              n4232 = call "CAN_Init-8.6.vi"("CAN卡类型"=w6082, "设备索引号"=w6083, "CAN端口"=w6084, "操作类型"=enum16{"初始化CAN", "关闭CAN"}."初始化CAN", "滤波方式"=w6087, "Accept Code"=u32 606601216, "簇"=T23 {"打开CAN"=FALSE, "初始化CAN"=TRUE, "开始CAN"=TRUE, "重启"=FALSE, "关闭CAN"=FALSE}, "Mask Code"=u32 524287 ("Accept Code"), "工作方式"=w6088, "是否滤波"=TRUE, "滤波选择"=T22 {"fiter_mode"=1, "fiter_endid"=75825152, "fiter_startid"=75890687}) -> ()  [unwired: 3 in, 6 out]
              n4233 = Wait Until Next ms Multiple(millisecond multiple=u32 20 ("毫秒倍数")) -> ()  [unwired: 1 out]
            }
            frame #1 {
              n4234 = local write "命令"(w6102) -> ()
              n4235 = call "ID组合.vi"("SA(4)"=0 ("PDU(1)"), "PS(3)"=63 ("PDU(1)"), "PF(2)"=w6102, "PDU(1)"=4) -> ("ID"=w6101:i32)  [unwired: 7 out]
              n4236 = local read "均衡类型选择"() -> (w6112:enum16{"放电均衡", "充电均衡", "充放电均衡"})
              n4237 = local write "命令序号"(3) -> ()
              n4238 = local read "设备索引号"() -> (w6107:u16)
              n4239 = local read "CAN卡类型"() -> (w6108:u32)
              n4240 = local read "CAN端口"() -> (w6106:u16)
              n4241 = Add(x=w6112, y=1) -> (x+y=w6110:i32)
              n4242 = Build Array(2, 3, w6110) -> (w6109:i32[])
              n4243 = call "transmit-8.6.vi"("can卡类型"=w6108, "设备索引号"=w6107, "CAN端口"=w6106, "ID"=w6101, "SendType"=u8 0, "Data"=w6109) -> ()  [unwired: 3 in, 11 out]
            }
            frame #2 {
              n4244 = Wait Until Next ms Multiple(millisecond multiple=u32 1000 ("毫秒倍数")) -> ()  [unwired: 1 out]
            }
            frame #3 {
              w6119 = u8 0 items=["Normal", "Listen Only"] ("工作方式")
              w6120 = u8 1 items=["Dual Filter", "Single Filter"] ("滤波方式")
              n4245 = local read "设备索引号"() -> (w6124:u16)
              n4246 = local read "CAN卡类型"() -> (w6125:u32)
              n4247 = global write "EV05全局变量1.vi" "流控帧 2"(FALSE ("流控帧 2")) -> ()
              n4248 = local read "CAN端口"() -> (w6123:u16)
              n4249 = local write "控制1"(FALSE ("控制1")) -> ()
              n4250 = local write "消除"(FALSE ("消除")) -> ()
